vi "VeriStand Launcher Utility.vi"   [LabVIEW 2014]
uses:
  NationalInstruments.VeriStand.Internal
panel:
  # "Launching NI VeriStand..."
types:
  T1 = enum32{"invalid app kind", "Development System", "Run Time System", "Student Edition", "Embedded LabVIEW", "Evaluation", "Custom"}
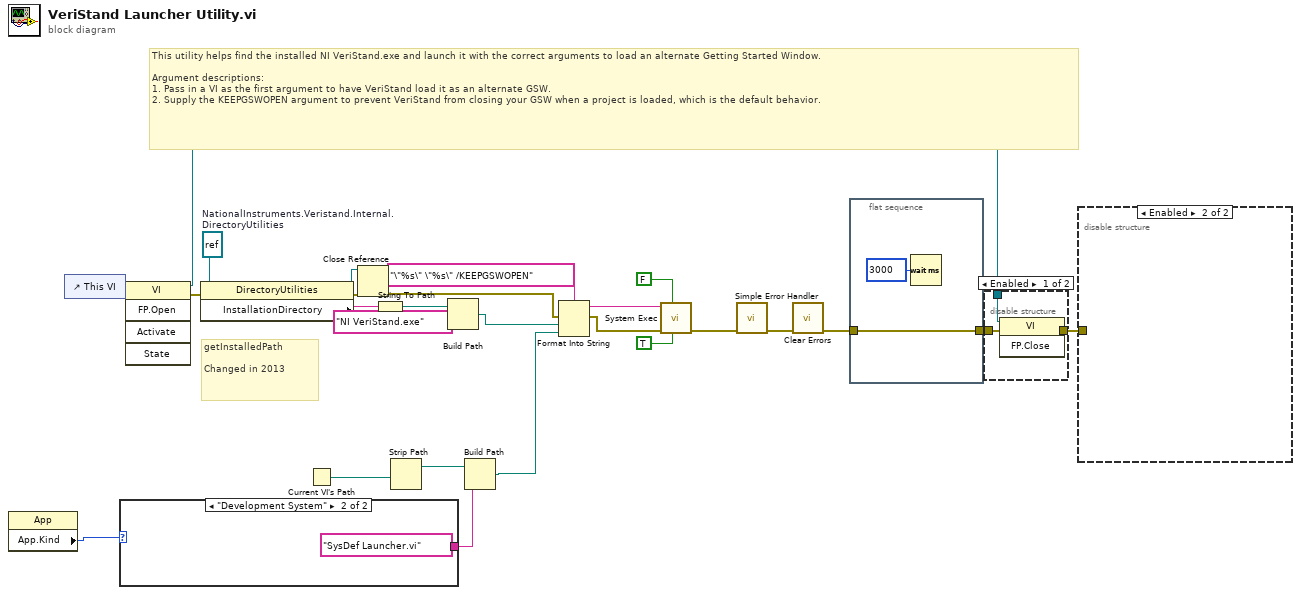
[diagram p0: block diagram]
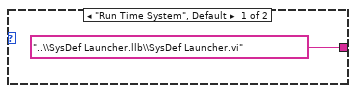
[diagram p2: hidden frame]
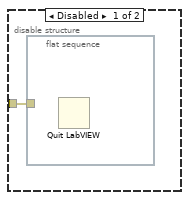
[diagram p4: hidden frame]
diagram:
  w13 = refnum<k24> refnum  # NationalInstruments.Veristand.Internal.DirectoryUtilities
  # "getInstalledPath\n\nChanged in 2013"
  # "This utility helps find the installed NI VeriStand.exe and launch it with the correct arguments to load an alternate Getting Started Window.\n\nArgument descriptions:\n1. Pass in a VI as the first argument to have VeriStand load it as an alternate GSW.\n2. Supply the KEEPGSWOPEN argument to prevent VeriStand from closing your GSW when a project is loaded, which is the default behavior."
  n1 = property class="App"() -> ("App.Kind"=w2:T1)  [unwired: 2 in, 2 out]
  n2 = control-ref of="This VI"() -> (w21:refnum<vi>)
  n3 = case shown="\"Development System\"" w2 {
    tunnel: ["..\\SysDef Launcher.llb\\SysDef Launcher.vi" ("Alternate GSW Name") "SysDef Launcher.vi" ("Alternate GSW Name")] -> w3
    frame "Run Time System", Default {
    }
    frame "Development System" {
    }
  }
  n4 = invoke class="VI" method="FP.Open"(reference=w21) -> (reference out=w10:refnum<vi>, error out=w12:errorcluster)  [unwired: 4 in, 3 out]
  n5 = property class="DirectoryUtilities"(reference=w13, error in=w12) -> (reference out=w8:refnum<k24>, error out=w9:errorcluster, "InstallationDirectory"=w11:string)
  n6 = Current VI's Path() -> (path=w5:path)
  n7 = Close Reference(reference=w8, error in (no error)=w9) -> (error out=w7:errorcluster)
  n8 = String To Path(string=w11) -> (path=w26:path)
  n9 = Strip Path(path=w5) -> (stripped path=w4:path)  [unwired: 1 out]
  n10 = Build Path(base path=w26, name or relative path="NI VeriStand.exe") -> (appended path=w23:path)
  n11 = Build Path(base path=w4, name or relative path=w3) -> (appended path=w1:path)
  n12 = Format Into String(format string="\"%s\" \"%s\" /KEEPGSWOPEN", error in=w7, w23, w1) -> (resulting string=w18:string, error out=w6:errorcluster)  [unwired: 1 in]
  n13 = call <vilib>:"System Exec.vi"("run minimized? (F)"=TRUE, "wait until completion? (T)"=FALSE, "error in (no error)"=w6, "command line"=w18) -> ("error out"=w22:errorcluster)  [unwired: 4 in, 3 out]
  n14 = call <vilib>:"Simple Error Handler.vi"("error in (no error)"=w22) -> ("error out"=w20:errorcluster)  [unwired: 4 in, 4 out]
  n15 = call <vilib>:"Clear Errors.vi"("error in (no error)"=w20) -> ("error out"=w15:errorcluster)  [unwired: 5 in, 1 out]
  n16 = flat-sequence {
    tunnel: w15 -> [w29]
    tunnel: [w29] -> w14
    frame #0 {
      n17 = Wait (ms)(milliseconds to wait=u32 3000) -> ()  [unwired: 1 out]
    }
  }
  n18 = disable-structure shown="Enabled" {
    disable-tunnel: [w33 _] -> w19
    disable-tunnel: w14 -> [w32 _]
    disable-tunnel: w10 -> [w31 _]
    frame Enabled {
      n19 = invoke class="VI" method="FP.Close"(reference=w31, error in=w32) -> (error out=w33:errorcluster)  [unwired: 1 in, 2 out]
    }
    frame Disabled {
    }
  }
  n20 = disable-structure shown="Enabled" {
    disable-tunnel: w19 -> [w34 _]
    frame Disabled {
      n21 = flat-sequence {
        tunnel: w34 -> [_]
        frame #0 {
          n22 = Quit LabVIEW() -> ()  [unwired: 1 in]
        }
      }
    }
    frame Enabled {
    }
  }
